vi "Stepper FPGA.vi"() -> ()   [LabVIEW 2012]
uses:
  <vilib>/rvi/eio/common/nirviEmuTemplateMethod_errors.vi
  <vilib>/eio/EIONode/EIONode.xnode
panel:
  out "Degrees (unlimited)":fxp<+/-,40,33>
  in  "Deg/Step":fxp<+,8,1>
  in  "Step Period":i16
  in  "Direction":bool
  in  "Enable/Disable":bool
  out "Step Period":i16
  in  "Stop":bool
  out "Pulses":fxp<+,18,17>
  out "Heartbeat":bool
  out "Degrees between 0 and 360":i32
  # "Motor Feedback"
  # "Motor Command"
  # "Calibrate Steps to Deg"
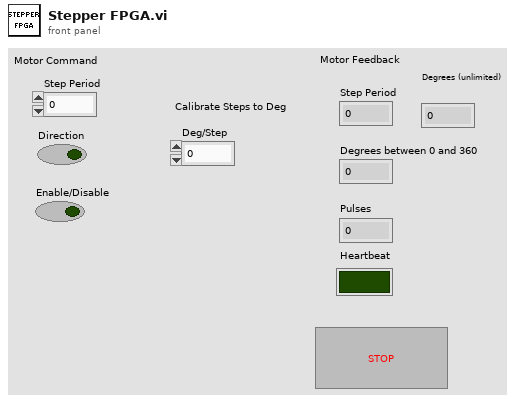
[diagram p1: front panel]
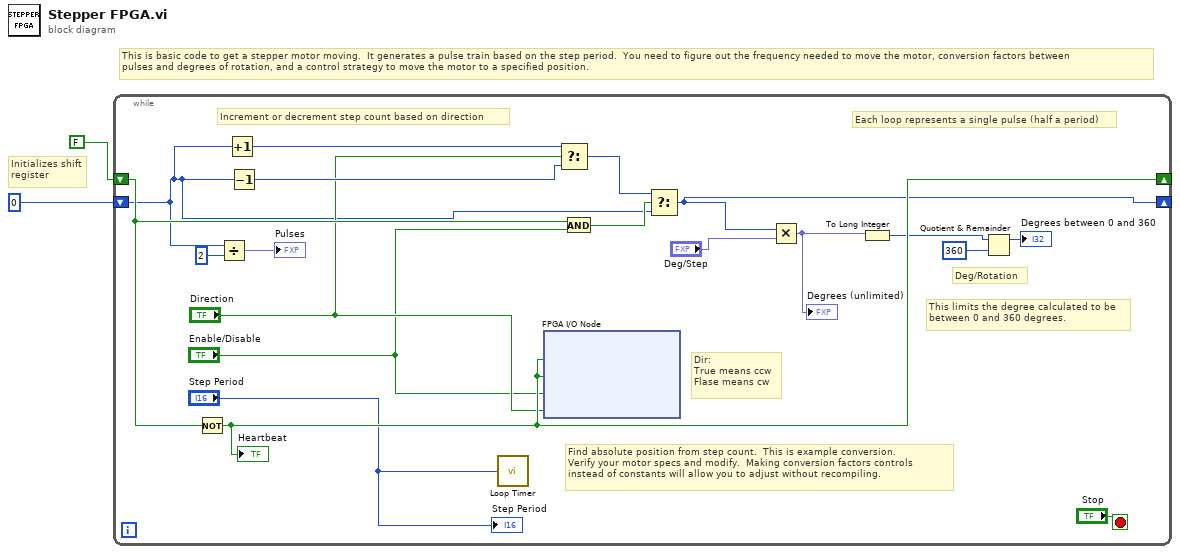
[diagram p0: block diagram]
diagram:
  # "Initializes shift\nregister"
  # "This is basic code to get a stepper motor moving.  It generates a pulse train based on the step period.  You need to figure out the frequency needed to move the motor, conversion factors between \npulses and degrees of rotation, and a control strategy to move the motor to a specified position."
  n1 = while {
    shift-right: [w12] -> _
    shift-left: 0 -> [w5]
    shift-right: [w19] -> _
    shift-left: FALSE -> [w20]
    stop <- "Stop" stop-if-true
    # "This limits the degree calculated to be\nbetween 0 and 360 degrees."
    # "Deg/Rotation"
    # "Each loop represents a single pulse (half a period)"
    # "Dir:\nTrue means ccw\nFlase means cw"
    # "Find absolute position from step count.  This is example conversion.  \nVerify your motor specs and modify.  Making conversion factors controls\ninstead of constants will allow you to adjust without recompiling."
    # "Increment or decrement step count based on direction"
    n2 = Not(x=w20) -> (.not. x?=w19:bool)
    "Heartbeat" <- w19
    n3 = Divide(x=w5, y=2) -> (x/y=→"Pulses":fxp<+/-,18,17>)
    n4 = Increment(x=w5) -> (x+1=w18:i32)
    n5 = Decrement(x=w5) -> (x-1=w17:i32)
    n6 = call "Loop Timer"("Count(uSec)"="Step Period") -> ()  [unwired: 1 out]
    n7 = xnode "FPGA I/O Node"("Stepper_Step"=w19, "Heartbeat LED"=w19, "Stepper_Enable"="Enable/Disable", "Stepper_Direction"="Direction") -> ()  [unwired: 4 in, 4 out]
    n8 = Select(t=w18, s="Direction", f=w17) -> (s? t:f=w16:i32)
    n9 = And(x=w20, y="Enable/Disable") -> (x .and. y?=w14:bool)
    n10 = Select(t=w16, s=w14, f=w5) -> (s? t:f=w12:i32)
    n11 = Multiply(x=w12, y="Deg/Step") -> (x*y=w6:fxp<+/-,40,33>)
    "Degrees (unlimited)" <- w6
    n12 = To Long Integer(number=w6) -> (32bit integer=w7:i32)
    n13 = Quotient & Remainder(x=w7, y=360) -> (x-y*floor(x/y)=→"Degrees between 0 and 360":i32)  [unwired: 1 out]
    "Step Period" <- "Step Period"
  }
